vi "Drive Reef Align_wrapper.vi"() -> ()   [LabVIEW 2023]
uses:
  <vilib>/Rock Robotics/WPI/Framework/Command Status Info.ctl
  <vilib>/Rock Robotics/WPI/Framework/Completion Status.ctl
  <vilib>/Rock Robotics/WPI/Framework/Completion Notifier.ctl
  swerve/Type Definitions/Data/Robot Velocities.ctl
  Implementation/Drive Operations.ctl
panel:
  in  "Auto Data":T2
  in  "Operation":T3=enum."Reef Align"
  in  "Angle Align":bool
  in  "Robot Velocities":T1
  in  "Left side":bool
  out "Command Info Out":T4
  in  "Description":string
  in  "Command Info In":T4
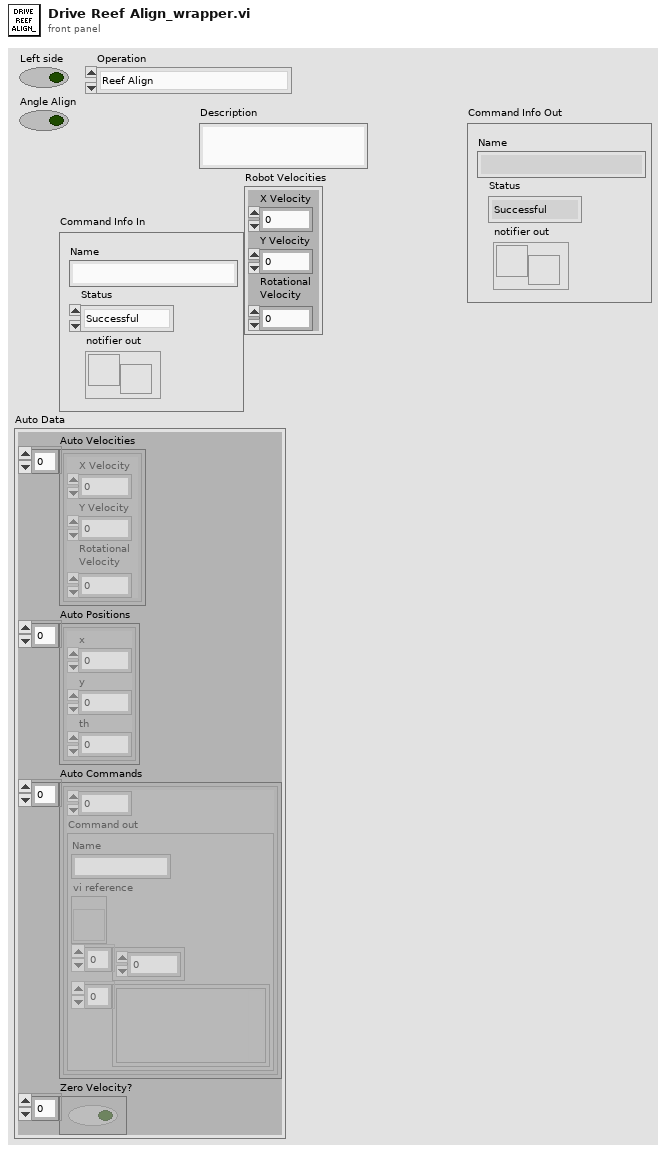
[diagram p1: front panel]
types:
  T1 = typedef "Robot Velocities.ctl" = cluster{"X Velocity":dbl, "Y Velocity":dbl, "Rotational \nVelocity":dbl}
  T2 = cluster{"Auto Velocities":T1[], "Auto Positions":cluster{"x":dbl, "y":dbl, "th":dbl}[], "Auto Commands":cluster{dbl, "Command out":cluster{"Name":string, "vi reference":refnum<vi>, i32[], variant[]}}[], "Zero Velocity?":bool[]}
  T3 = typedef "Drive Operations.ctl" = enum16{"Reserve", "Read Current", "Immediate", "Calibrate", "Reef Align", "Auto"}
  T4 = typedef "Command Status Info.ctl" = cluster{"Name":string, "Status":T5, "notifier out":T6}
  T5 = typedef "Completion Status.ctl" = enum16{"Successful", "Aborted", "Incomplete"}
  T6 = typedef "Completion Notifier.ctl" = refnum<notifier>
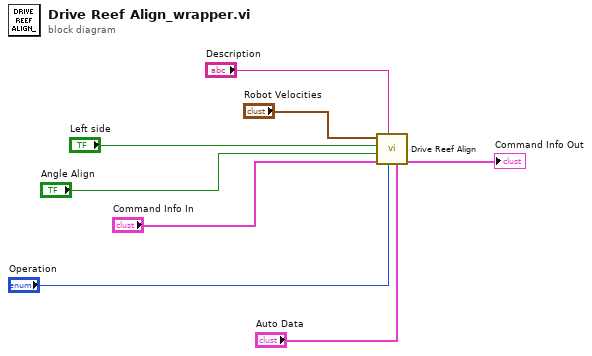
[diagram p0: block diagram]
diagram:
  n1 = call "Drive Reef Align.vi"("Auto Data"="Auto Data", "Operation"="Operation", "Description"="Description", "Command Info In"="Command Info In", "Angle Align"="Angle Align", "Left Side?"="Left side", "Robot Velocities"="Robot Velocities") -> ("Command Info Out"=→"Command Info Out":T4)  [unwired: 4 in]
